vi "Copy of VISA_IDN.vi"(0 "Session In":refnum<visa-resource-name>="TCPIP0::10.0.1.24::inst0::INSTR", 5 "error in":errorcluster {"code" format="%.0x"}) -> (13 "concatenated string":string, 14 "Session Out":refnum<visa-resource-name>, 15 "Mfr":string, 16 "Model":string, 17 "Ver":string, 18 "SN":string, 19 "error out":errorcluster {"code" format="%.0x"})   [LabVIEW 2018]
panel:
  out "Address":string
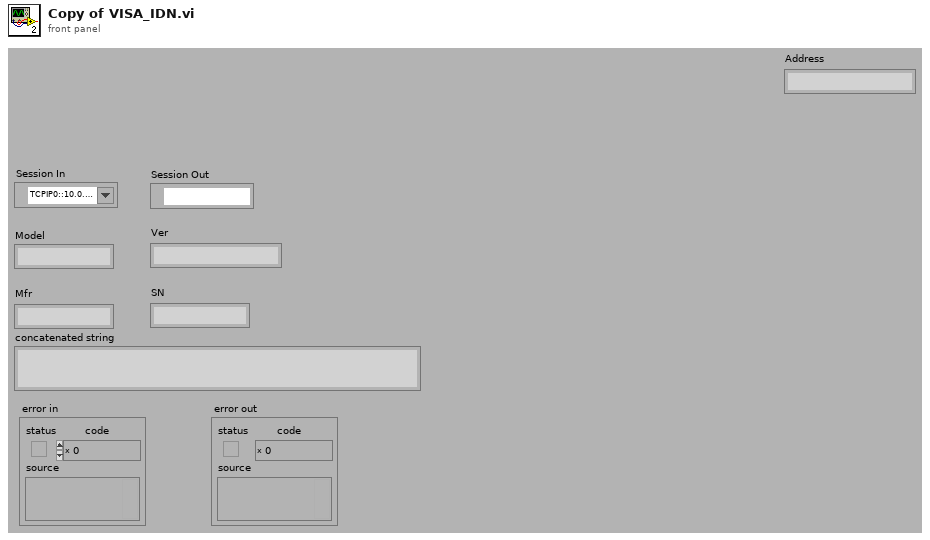
[diagram p1: front panel]
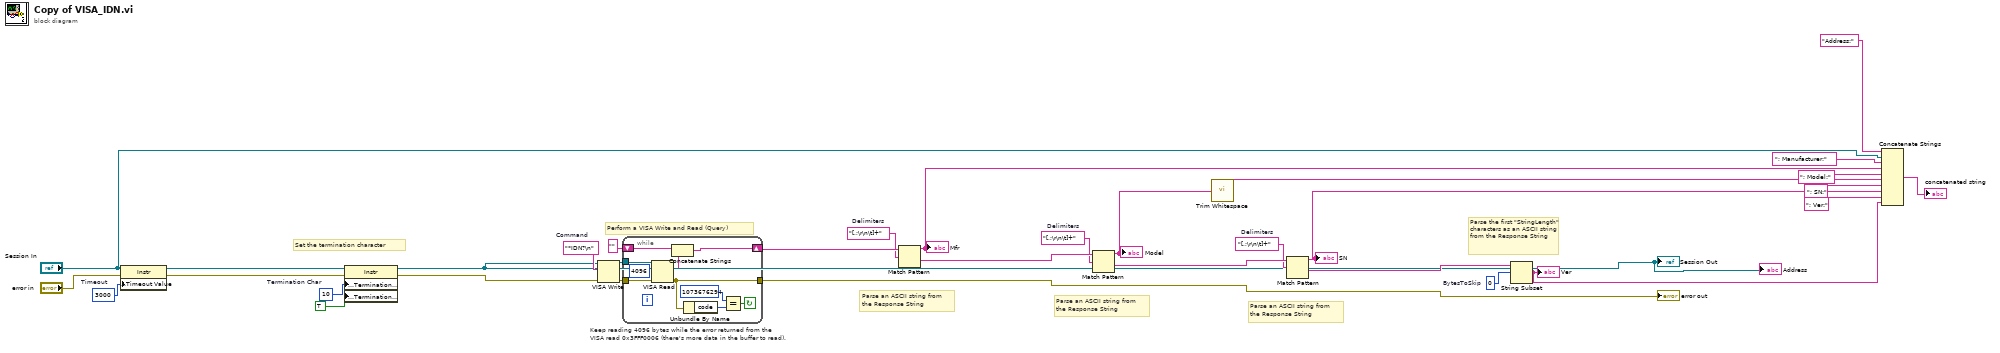
[diagram p0: block diagram]
diagram:
  w14 = 0  # BytesToSkip
  w15 = "[,;\r\n\t]+"  # Delimiters
  w17 = "[,;\r\n\t]+"  # Delimiters
  w19 = "[,;\r\n\t]+"  # Delimiters
  w21 = "*IDN?\n"  # Command
  w28 = u8 10  # Termination Char
  w33 = u32 3000  # Timeout
  # "Parse the first \"StringLength\" characters as an ASCII string from the Response String"
  # "Parse an ASCII string from the Response String"
  # "Parse an ASCII string from the Response String"
  # "Parse an ASCII string from the Response String"
  # "Perform a VISA Write and Read (Query)"
  # "Keep reading 4096 bytes while the error returned from the\nVISA read 0x3FFF0006 (there's more data in the buffer to read)."
  # "Set the termination character"
  n1 = property class="Instr"(reference="Session In", error in="error in", "General Settings:Timeout Value"=w33) -> (reference out=w31:refnum<visa-resource-name>, error out=w30:errorcluster)
  n2 = property class="Instr"(reference=w31, error in=w30, "Message Based Settings:Termination Character"=w28, "Message Based Settings:Termination Character Enable"=TRUE ("enable")) -> (reference out=w10:refnum<visa-resource-name>, error out=w29:errorcluster)
  "Session Out" <- w10
  "Address" <- w10
  n3 = VISA Write(VISA resource name=w10, write buffer=w21, error in (no error)=w29) -> (VISA resource name out=w26:refnum<visa-resource-name>, error out=w24:errorcluster)  [unwired: 1 out]
  n4 = while {
    tunnel: w26 -> [w40]
    shift-right: [w34] -> w25
    shift-left: "" -> [w39]
    tunnel: w24 -> [w37]
    tunnel: [w36] -> w23
    stop <- w35 continue-if-true
    n5 = VISA Read(VISA resource name=w40, byte count=u32 4096 ("byte count (0)"), error in (no error)=w37) -> (read buffer=w38:string, error out=w36:errorcluster)  [unwired: 2 out]
    n6 = Concatenate Strings(w39, w38) -> (w34:string)
    n7 = Unbundle By Name(w36) -> ("code"=w42:i32)
    n8 = Equal?(x=1073676294, y=w42) -> (x = y?=w35:bool)
  }
  "error out" <- w23
  n9 = Match Pattern(string=w25, regular expression=w19) -> (before substring=w8:string, after substring=w20:string)  [unwired: 1 in, 2 out]
  "Mfr" <- w8
  n10 = Match Pattern(string=w20, regular expression=w17) -> (before substring=w13:string, after substring=w18:string)  [unwired: 1 in, 2 out]
  "Model" <- w13
  n11 = call <vilib>:"Trim Whitespace.vi"("string"=w13) -> ("trimmed string"=w6:string)  [unwired: 1 in]
  n12 = Match Pattern(string=w18, regular expression=w15) -> (before substring=w4:string, after substring=w16:string)  [unwired: 1 in, 2 out]
  "SN" <- w4
  n13 = String Subset(string=w16, offset (0)=w14) -> (substring=w2:string)  [unwired: 1 in]
  "Ver" <- w2
  n14 = Concatenate Strings("Address:" ("string"), "Session In", "; Manufacturer:", w8, "; Model:", w6, "; SN:" ("string"), w4, "; Ver:" ("string"), w2) -> (→"concatenated string":string)
